vi "Begin.vi"(8 "error in (no error)":errorcluster, 11 "Dev Motors with Brake in":refnum<class "Dev Motors with Brake.lvclass">) -> (0 "error out":errorcluster, 3 "Dev Motors with Brake out":refnum<class "Dev Motors with Brake.lvclass">)   [LabVIEW 2014, in "Dev Motors with Brake.lvlib" / "Dev Motors with Brake.lvclass"]
uses:
  Dev Motors with Brake.lvclass
  Dev Motors with Brake.lvclass/Dev Motors with Brake.ctl
  <vilib>/Rock Robotics/WPI/Solenoid/WPI_SolenoidOpenDouble.vi
  Comp Robot/Comp Motors with Encoders/Comp Motors with Encoders Class/Comp Motors with Encoders.lvclass
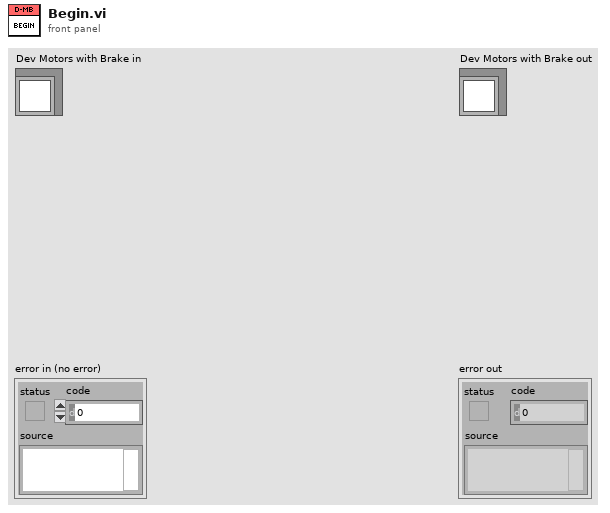
[diagram p1: front panel]
types:
  T1 = typedef "WPI_SolenoidChannel.ctl" = enum8{"Solenoid 0", "Solenoid 1", "Solenoid 2", "Solenoid 3", "Solenoid 4", "Solenoid 5", "Solenoid 6", "Solenoid 7", "Invalid"}
  T2 = typedef "WPI_SolenoidDevRef.ctl" = cluster{"DevStatus":errorcluster, "Pneumatics Control Module":u8, "Forward Solenoid Channel":T1, "Reverse Solenoid Channel":T1}
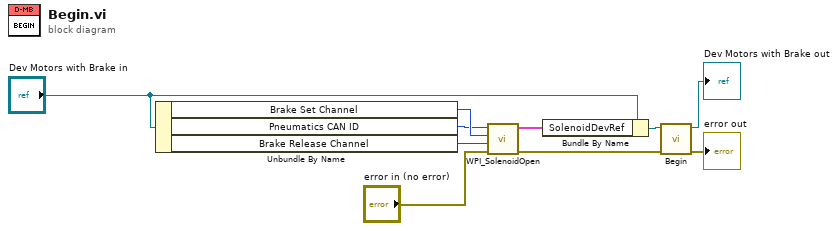
[diagram p0: block diagram]
diagram:
  n1 = Unbundle By Name("Dev Motors with Brake in") -> ("Brake Set Channel"=w7:T1, "Pneumatics CAN ID"=w5:u8, "Brake Release Channel"=w6:T1)
  n2 = call-poly <vilib>:"WPI_SolenoidOpen.vi"("error in (no error)"="error in (no error)", "Reverse Solenoid Channel"=w6, "Forward Solenoid Channel"=w7, "Pneumatics Control Module (0)"=w5) -> ("error out"=w1:errorcluster, "SolenoidDevRef"=w3:T2)  [unwired: 6 in]
  n3 = Bundle By Name(cluster="Dev Motors with Brake in", "SolenoidDevRef"=w3) -> (w4:refnum<class "Dev Motors with Brake.lvclass">)
  n4 = call-parent "Begin.vi"("error in (no error)"=w1, "Comp Motors with Encoders in"=w4) -> ("error out"=→"error out":errorcluster, "Comp Motors with Encoders out"=→"Dev Motors with Brake out":refnum<class "Dev Motors with Brake.lvclass">)  [unwired: 8 in]
